vi "libzmq32 path.vi"() -> (2 "path":path)   [LabVIEW 2019, in "RemoteControl.ZMQ.lvlib" / "libzmq32.lvclass"]
uses:
  libzmq32.lvclass
  <vilib>/addons/zeromq/zeromq.lvlib
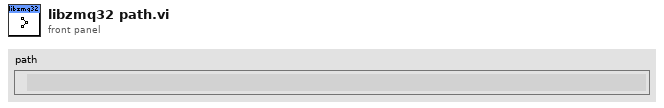
[diagram p1: front panel]
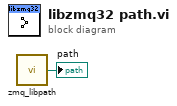
[diagram p0: block diagram]
diagram:
  n1 = call <vilib>:"zmq_libpath.vi"() -> ("path"=→"path":path)
